vi "DHE_SetPixWriteTimeAlgors.vi"(2 "write_pix_time_algors":string) -> ()   [LabVIEW 2016]
uses:
  private/vis/DHE_VarAction.ctl
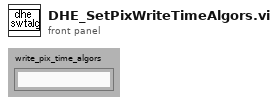
[diagram p1: front panel]
types:
  T1 = typedef "DHE_VarAction.ctl" = enum16{"read", "write"}
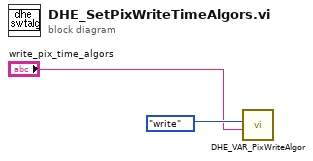
[diagram p0: block diagram]
diagram:
  n1 = call "DHE_VAR_PixWriteAlgor.vi"("value"="write_pix_time_algors", "action"=DHE_VarAction."write") -> ()  [unwired: 10 out]
